vi "난수플롯이벤트.vi"() -> ()   [LabVIEW 2018]
panel:
  in  "정지":bool
  out "웨이브폼 차트":dbl(graph)
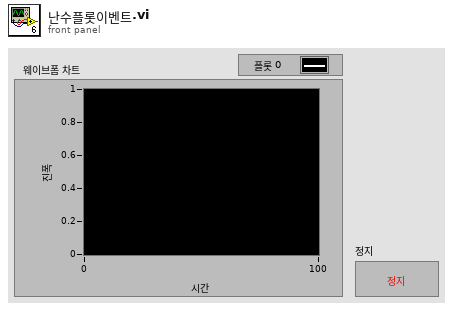
[diagram p1: front panel]
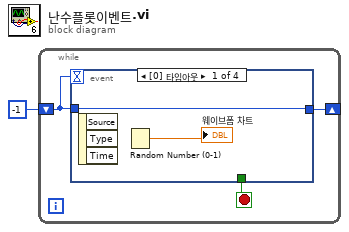
[diagram p0: block diagram]
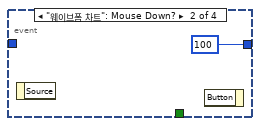
[diagram p2: hidden frame]
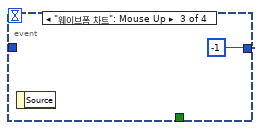
[diagram p3: hidden frame]
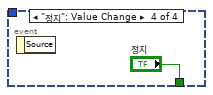
[diagram p4: hidden frame]
diagram:
  n1 = while {
    shift-right: [w4] -> _
    shift-left: -1 -> [w3]
    stop <- w2 stop-if-true
    n2 = event shown="[0] 타임아웃" {
      selector: _ -> [_ _ _ _]
      dyn-events: _ -> [_ _ _ _]
      timeout: w3 -> [_ _ _ _]
      tunnel: w3 -> [w6 _ _ _]
      tunnel: [w6 100 -1 _] -> w4
      tunnel: [_ _ _ "정지"] -> w2
      event Timeout {
        n3 = event-data() -> ()  [unwired: 1 in, 3 out]
        n4 = Random Number (0-1)() -> (number: 0 to 1=→"웨이브폼 차트":dbl)
      }
      event "웨이브폼 차트": Mouse Down? {
        n5 = event-data() -> ()  [unwired: 1 in, 1 out]
        n6 = event-data() -> ()  [unwired: 2 in, 1 out]
      }
      event "웨이브폼 차트": Mouse Up {
        n7 = event-data() -> ()  [unwired: 1 in, 1 out]
      }
      event "정지": Value Change {
        n8 = event-data() -> ()  [unwired: 1 in, 1 out]
      }
    }
  }
